vi "I2C.vi"(9 "I2C[37:0]_READ":bool[](array[boolean])=[FALSE, TRUE, FALSE, TRUE, TRUE, TRUE, FALSE, FALSE, FALSE, FALSE, FALSE, FALSE, FALSE, FALSE, FALSE, FALSE, FALSE, FALSE, TRUE, FALSE, FALSE, TRUE, FALSE, TRUE, TRUE, TRUE, FALSE, TRUE, FALSE, FALSE, FALSE, FALSE, FALSE, FALSE, FALSE, FALSE, FALSE, FALSE], 10 "I2C[26:0]_WRITE":bool[](array[boolean])=[FALSE, TRUE, FALSE, TRUE, TRUE, TRUE, FALSE, FALSE, FALSE, FALSE, FALSE, FALSE, FALSE, FALSE, FALSE, FALSE, FALSE, FALSE, FALSE, FALSE, FALSE, FALSE, FALSE, FALSE, FALSE, FALSE, FALSE], 11 "R(T)/W(F)":bool) -> (3 "DATA":bool[](array[boolean]))   [LabVIEW 2018]
uses:
  <vilib>/Platform/TimedLoop/XDataNode/timing_clust.ctl
  <vilib>/Platform/TimedLoop/XDataNode/nitl_modes.ctl
  <vilib>/Platform/TimedLoop/XDataNode/wakeup.ctl
  <vilib>/rvi/Emulation/niFpgaSctlEmulationGetInTimedLoop.vi
  <vilib>/rvi/Emulation/niFpgaEmulationReportErrorSimple.vi
  <vilib>/rvi/Emulation/niFpgaGetClockAttributes.vi
  <vilib>/rvi/Emulation/niFpgaCriticalErrorInLSC.vi
  <vilib>/rvi/eio/common/nirviEmuTemplateMethod_errors.vi
  <vilib>/Platform/TimedLoop/XDataNode/XDataNode.xnode
  <vilib>/eio/EIONode/EIONode.xnode
  <vilib>/Platform/TimedLoop/XDataNode/XDNodeRunTimeDep.lvlib
panel:
  # "Если SERADD равен 0, то ниже верная последовательность."
  # "6"
  # "5"
  # "4"
  # "3"
  # "2"
  # "1"
  # "0"
  # "W"
  # "WACK"
  # "7"
  # "6"
  # "5"
  # "4"
  # "3"
  # "2"
  # "1"
  # "0"
  # "WACK"
  # "7"
  # "6"
  # "5"
  # "4"
  # "3"
  # "2"
  # "1"
  # "0"
  # "WACK"
  # "6"
  # "5"
  # "4"
  # "3"
  # "2"
  # "1"
  # "0"
  # "W"
  # "WACK"
  # "7"
  # "6"
  # "5"
  # "4"
  # "3"
  # "2"
  # "1"
  # "0"
  # "WACK"
  # "\"1\""
  # "6"
  # "5"
  # "4"
  # "3"
  # "2"
  # "1"
  # "0"
  # "R"
  # "\"0\""
  # "WACK"
  # "7"
  # "6"
  # "5"
  # "4"
  # "3"
  # "2"
  # "1"
  # "0"
  # "RACK"
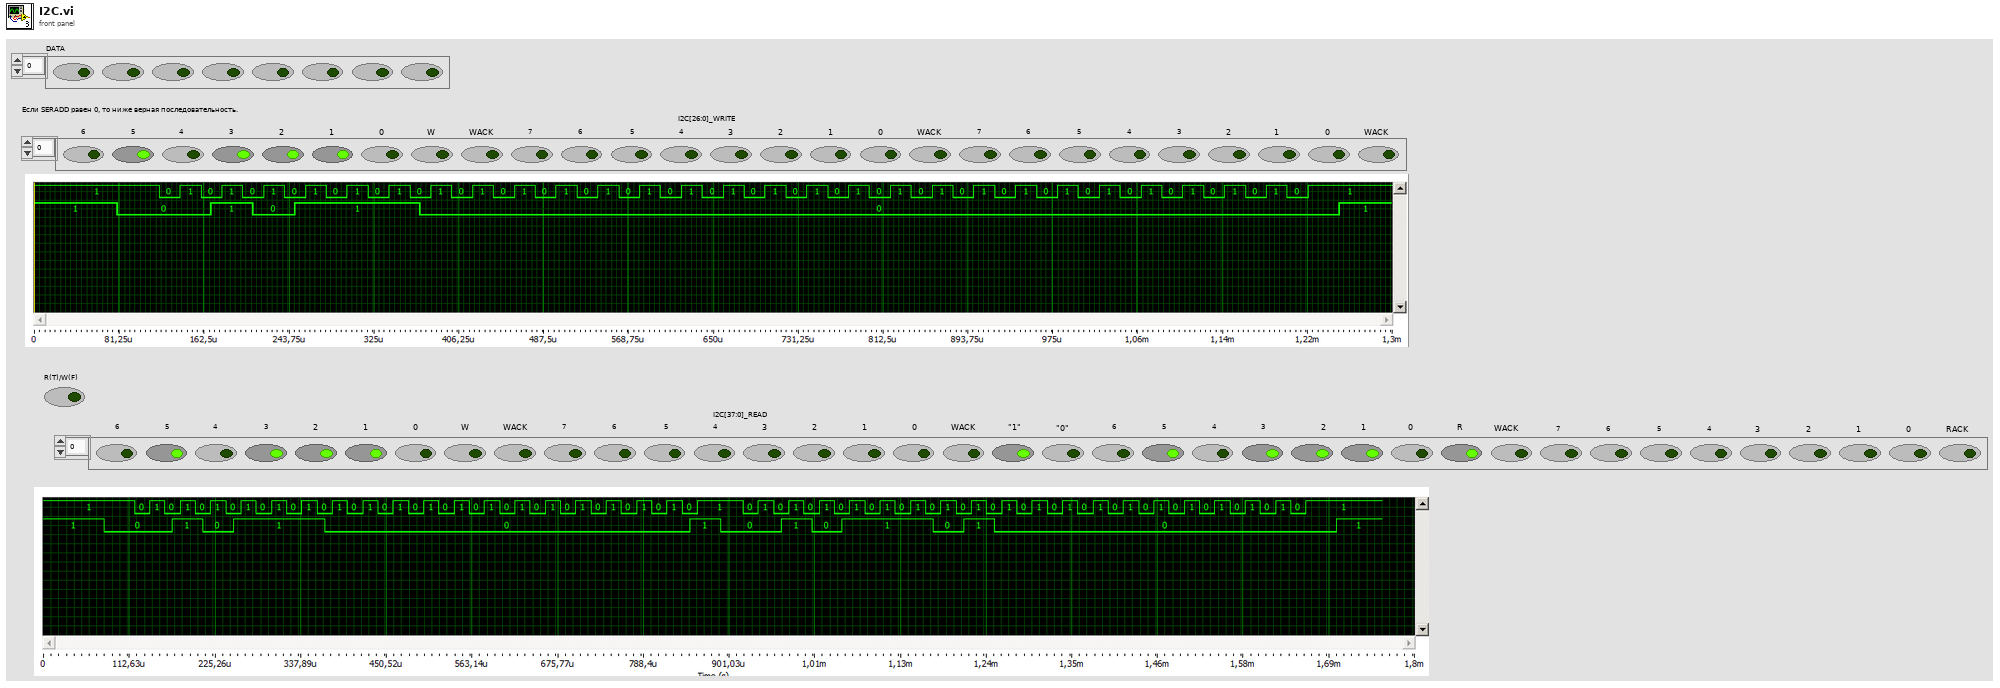
[diagram p1: front panel]
types:
  T1 = typedef "XDNodeRunTimeDep.lvlib/timing_clust.ctl" = cluster{"Expected End [f-1]":u64, "Actual End [f-1]":u64, "Finished Late? [f-1]":bool, "Expected End [i-1]":u64, "Actual End [i-1]":u64, "Finished Late? [i-1]":bool, "Expected Start [i]":u64, "Actual Start [i]":u64, "Expected Start [f]":u64, "Actual Start [f]":u64, "Source Name":string, "Structure Name":string, "Period":i64, "Deadline":i64, "Offset":i64, "Start":i64, "Priority":i32, "Timeout":i32, "Mode":T2, "Wakeup Reason":T3, "Error":errorcluster, "Source Type":string, "Secondary Source Type":string, "Global End Time":u64, "Global Start Time":u64, "Frame Duration":u64, "Iteration Duration":u64, "Assigned CPU":i32, "I/O Scan Engine Mode":u32}
  T2 = typedef "XDNodeRunTimeDep.lvlib/nitl_modes.ctl" = enum32{"No Change", "Process missed periods, maintain original phase", "Discard missed periods, maintain original phase", "Process missed periods, ignore original phase", "Discard missed periods, ignore original phase"}
  T3 = typedef "XDNodeRunTimeDep.lvlib/wakeup.ctl" = enum32{"Normal", "Aborted", "Asynchronous wakeup", "Timing source error", "Timed loop error", "Timeout"}
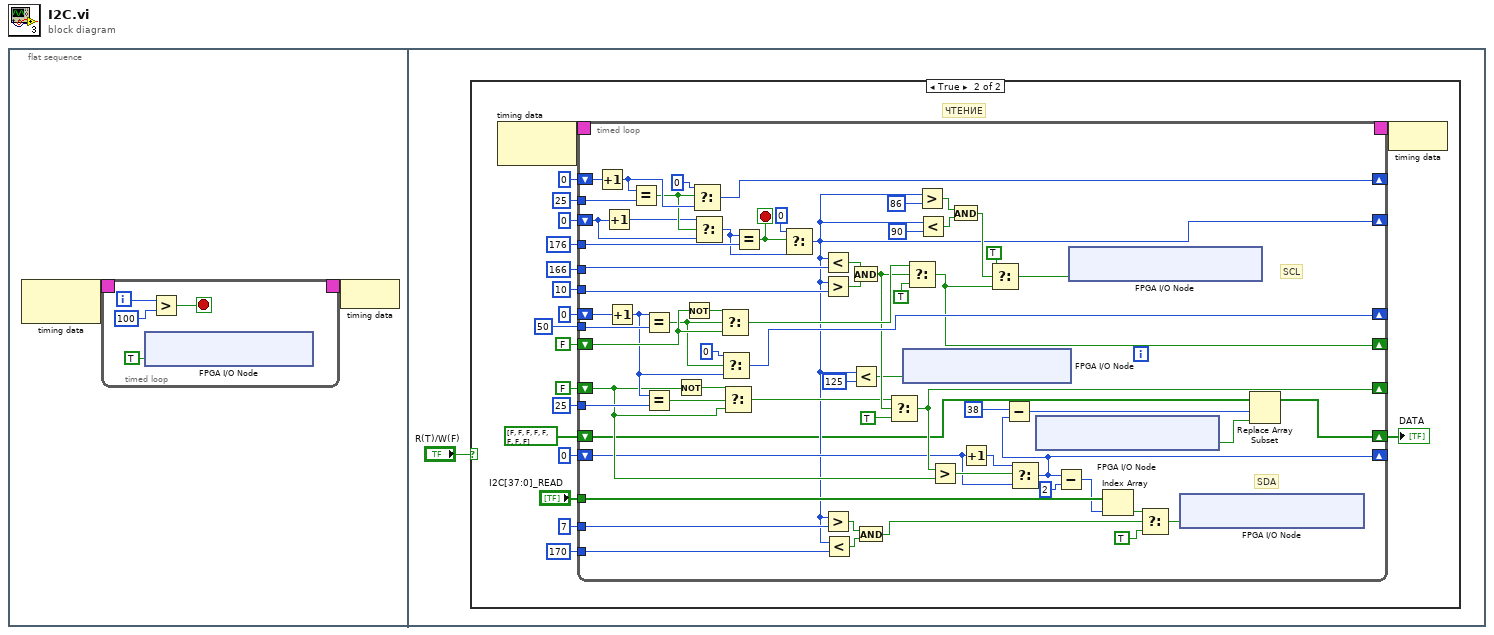
[diagram p0: block diagram]
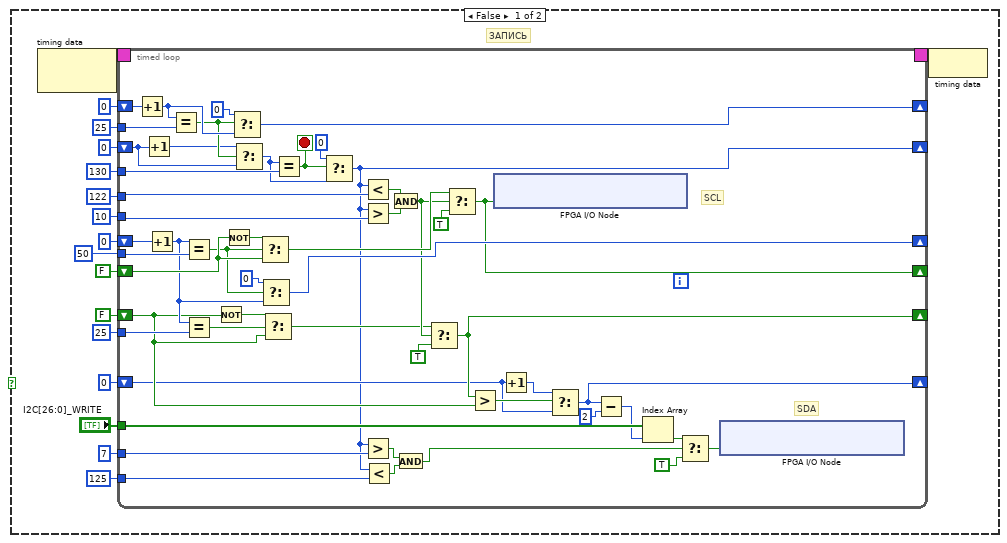
[diagram p2: hidden frame]
diagram:
  n1 = flat-sequence {
    frame #0 {
      n2 = node-c288() -> (w2:T1)  [unwired: 1 in]
      n3 = timed-loop {
        timing: w2 -> [_]
        timing-out: [_] -> w1
        i -> [w5]
        stop <- w3 stop-if-true
        n4 = xnode "FPGA I/O Node"("IO Module\\DDCA_PFI_WE"=TRUE ("IO Module\\DDCA_PFI_WE")) -> ()  [unwired: 1 in, 1 out]
        n5 = Greater?(x=w5, y=u8 100 ("x")) -> (0:w3:bool)
      }
      n6 = node-c288(w1) -> ()
    }
    frame #1 {
      n7 = case shown="True" "R(T)/W(F)" {
        frame False {
          # "ЗАПИСЬ"
          n8 = node-c288() -> (w28:T1)  [unwired: 1 in]
          n9 = timed-loop {
            timing: w28 -> [_]
            timing-out: [_] -> w27
            tunnel: u8 7 ("8") -> [w40]
            tunnel: u8 10 ("10") -> [w59]
            tunnel: u8 122 ("122") -> [w60]
            tunnel: u8 25 ("25") -> [w78]
            shift-right: [w72] -> _
            shift-left: u8 0 -> [w79]
            shift-right: [w33] -> _
            shift-left: u8 0 -> [w73]
            tunnel: u8 130 ("130") -> [w71]
            shift-right: [w61] -> _
            shift-left: u8 0 -> [w67]
            tunnel: u8 50 ("50") -> [w66]
            shift-right: [w54] -> _
            shift-left: FALSE -> [w65]
            shift-right: [w46] -> _
            shift-left: FALSE -> [w45]
            tunnel: u8 25 ("50") -> [w52]
            shift-right: [w36] -> _
            shift-left: u8 0 -> [w41]
            tunnel: "I2C[26:0]_WRITE" -> [w42]
            tunnel: u8 125 ("122") -> [w30]
            stop <- w68 stop-if-true
            # "SDA"
            # "SCL"
            n10 = Increment(x=w79) -> (x+1=w76:u8)
            n11 = Increment(x=w73) -> (x+1=w74:u8)
            n12 = Increment(x=w67) -> (x+1=w53:u8)
            n13 = Equal?(x=w76, y=w78) -> (x = y?=w75:bool)
            n14 = Equal?(x=w53, y=w66) -> (x = y?=w63:bool)
            n15 = Equal?(x=w53, y=w52) -> (x = y?=w51:bool)
            n16 = Not(x=w45) -> (.not. x?=w50:bool)
            n17 = Not(x=w65) -> (.not. x?=w64:bool)
            n18 = Select(t=u8 0, s=w75, f=w76) -> (s? t:f=w72:u8)
            n19 = Select(t=w74, s=w75, f=w73) -> (s? t:f=w69:u8)
            n20 = Select(t=w64, s=w63, f=w65) -> (s? t:f=w56:bool)
            n21 = Select(t=u8 0, s=w63, f=w53) -> (s? t:f=w61:u8)
            n22 = Select(t=w50, s=w51, f=w45) -> (s? t:f=w47:bool)
            n23 = Equal?(x=w69, y=w71) -> (x = y?=w68:bool)
            n24 = Select(t=u8 0, s=w68, f=w69) -> (s? t:f=w33:u8)
            n25 = Less?(x=w33, y=w60) -> (x < y?=w58:bool)
            n26 = Greater?(x=w33, y=w59) -> (0:w57:bool)
            n27 = Greater?(x=w33, y=w40) -> (0:w31:bool)
            n28 = Less?(x=w33, y=w30) -> (x < y?=w32:bool)
            n29 = And(x=w58, y=w57) -> (x .and. y?=w48:bool)
            n30 = And(x=w31, y=w32) -> (x .and. y?=w29:bool)
            n31 = Select(t=w47, s=w48, f=TRUE) -> (s? t:f=w46:bool)
            n32 = Select(t=w56, s=w48, f=TRUE) -> (s? t:f=w54:bool)
            n33 = Greater?(x=w46, y=w45) -> (0:w44:bool)
            n34 = xnode "FPGA I/O Node"("IO Module\\DDCA_DIO21_Write"=w54) -> ()  [unwired: 1 in, 1 out]
            n35 = Increment(x=w41) -> (x+1=w43:u8)
            n36 = Select(t=w43, s=w44, f=w41) -> (s? t:f=w36:u8)
            n37 = Subtract(x=w36, y=u8 2) -> (x-y=w34:u8)
            n38 = Index Array(array=w42, index=w34) -> (element=w38:bool)
            n39 = Select(t=w38, s=w29, f=TRUE) -> (s? t:f=w37:bool)
            n40 = xnode "FPGA I/O Node"("IO Module\\DDCA_PFI1_Write"=w37) -> ()  [unwired: 1 in, 1 out]
          }
          n41 = node-c288(w27) -> ()
        }
        frame True {
          # "ЧТЕНИЕ"
          n42 = node-c288() -> (w102:T1)  [unwired: 1 in]
          n43 = timed-loop {
            timing: w102 -> [_]
            timing-out: [_] -> w101
            tunnel: u8 7 ("8") -> [w129]
            tunnel: u8 10 ("10") -> [w147]
            tunnel: u8 166 ("122") -> [w148]
            tunnel: u8 25 ("25") -> [w166]
            shift-right: [w160] -> _
            shift-left: u8 0 -> [w167]
            shift-right: [w111] -> _
            shift-left: u8 0 -> [w161]
            tunnel: u8 176 ("130") -> [w159]
            shift-right: [w149] -> _
            shift-left: u8 0 -> [w155]
            tunnel: u8 50 ("50") -> [w154]
            shift-right: [w118] -> _
            shift-left: FALSE -> [w153]
            shift-right: [w135] -> _
            shift-left: FALSE -> [w134]
            tunnel: u8 25 ("50") -> [w141]
            shift-right: [w108] -> _
            shift-left: u8 0 -> [w130]
            tunnel: "I2C[37:0]_READ" -> [w131]
            tunnel: u8 170 ("122") -> [w121]
            shift-right: [w105] -> w84
            shift-left: bool[] [FALSE, FALSE, FALSE, FALSE, FALSE, FALSE, FALSE, FALSE] ("DATA") -> [w106]
            stop <- w156 stop-if-true
            # "SDA"
            # "SCL"
            n44 = Increment(x=w167) -> (x+1=w164:u8)
            n45 = Increment(x=w161) -> (x+1=w162:u8)
            n46 = Increment(x=w155) -> (x+1=w142:u8)
            n47 = Equal?(x=w164, y=w166) -> (x = y?=w163:bool)
            n48 = Equal?(x=w142, y=w154) -> (x = y?=w151:bool)
            n49 = Equal?(x=w142, y=w141) -> (x = y?=w140:bool)
            n50 = Not(x=w134) -> (.not. x?=w139:bool)
            n51 = Not(x=w153) -> (.not. x?=w152:bool)
            n52 = Select(t=u8 0, s=w163, f=w164) -> (s? t:f=w160:u8)
            n53 = Select(t=w162, s=w163, f=w161) -> (s? t:f=w157:u8)
            n54 = Select(t=w152, s=w151, f=w153) -> (s? t:f=w144:bool)
            n55 = Select(t=u8 0, s=w151, f=w142) -> (s? t:f=w149:u8)
            n56 = Select(t=w139, s=w140, f=w134) -> (s? t:f=w136:bool)
            n57 = Equal?(x=w157, y=w159) -> (x = y?=w156:bool)
            n58 = Select(t=u8 0, s=w156, f=w157) -> (s? t:f=w111:u8)
            n59 = Less?(x=w111, y=w148) -> (x < y?=w146:bool)
            n60 = Greater?(x=w111, y=w147) -> (0:w145:bool)
            n61 = Greater?(x=w111, y=w129) -> (0:w122:bool)
            n62 = Less?(x=w111, y=w121) -> (x < y?=w123:bool)
            n63 = And(x=w146, y=w145) -> (x .and. y?=w137:bool)
            n64 = Less?(x=w111, y=u8 125) -> (x < y?=w103:bool)
            n65 = And(x=w122, y=w123) -> (x .and. y?=w120:bool)
            n66 = Select(t=w136, s=w137, f=TRUE) -> (s? t:f=w135:bool)
            n67 = xnode "FPGA I/O Node"("IO Module\\DDCA_PFI_WE"=w103) -> ()  [unwired: 1 in, 1 out]
            n68 = Select(t=w144, s=w137, f=TRUE) -> (s? t:f=w118:bool)
            n69 = Greater?(x=w111, y=u8 86) -> (0:w116:bool)
            n70 = Less?(x=w111, y=u8 90) -> (x < y?=w117:bool)
            n71 = Greater?(x=w135, y=w134) -> (0:w133:bool)
            n72 = And(x=w116, y=w117) -> (x .and. y?=w115:bool)
            n73 = Increment(x=w130) -> (x+1=w132:u8)
            n74 = Select(t=TRUE, s=w115, f=w118) -> (s? t:f=w119:bool)
            n75 = Select(t=w132, s=w133, f=w130) -> (s? t:f=w108:u8)
            n76 = Subtract(x=u8 38 ("50"), y=w108) -> (x-y=w107:u8)
            n77 = xnode "FPGA I/O Node"() -> ("IO Module\\DDCA_PFI1_Read"=w104:bool)  [unwired: 1 in, 1 out]
            n78 = Subtract(x=w108, y=u8 2) -> (x-y=w124:u8)
            n79 = xnode "FPGA I/O Node"("IO Module\\DDCA_DIO21_Write"=w119) -> ()  [unwired: 1 in, 1 out]
            n80 = Index Array(array=w131, index=w124) -> (element=w127:bool)
            n81 = Select(t=w127, s=w120, f=TRUE) -> (s? t:f=w126:bool)
            n82 = xnode "FPGA I/O Node"("IO Module\\DDCA_PFI1_Write"=w126) -> ()  [unwired: 1 in, 1 out]
            n83 = Replace Array Subset(array=w106, new element=w104, index=w107) -> (w105:bool[])
          }
          "DATA" <- w84
          n84 = node-c288(w101) -> ()
        }
      }
    }
  }
